vi "Const_uitlity.vi"(1 "Duration":dbl format="%#_13g") -> (0 "Minutes passed":dbl format="%#_13g")   [LabVIEW 2016]
uses:
  Global/Global Variables/Data_Display_global.vi
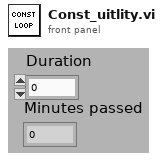
[diagram p1: front panel]
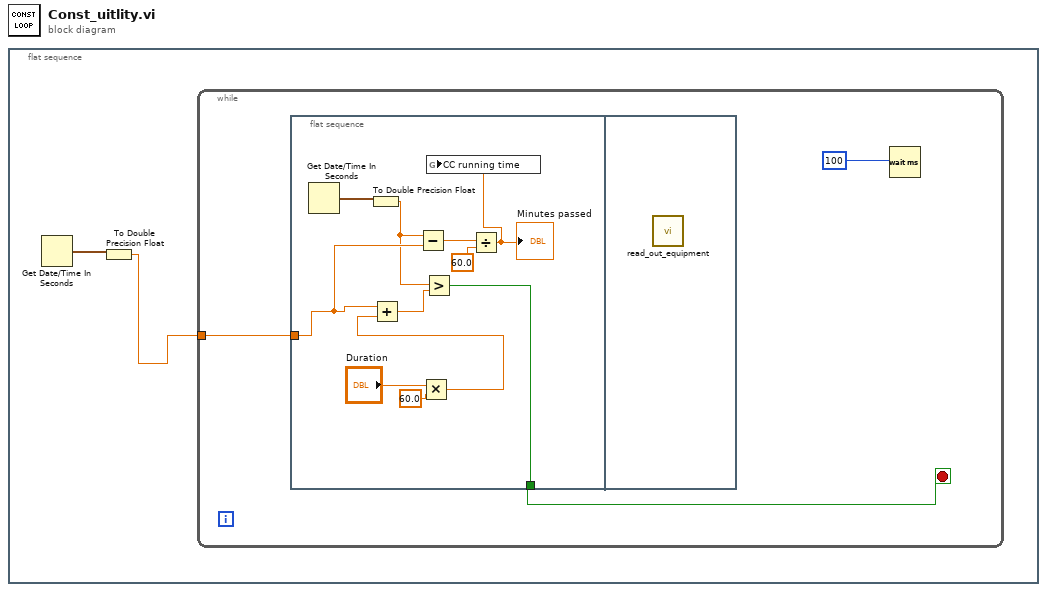
[diagram p0: block diagram]
diagram:
  n1 = flat-sequence {
    frame #0 {
      n2 = Get Date/Time In Seconds() -> (seconds since 1Jan1904=w2:timestamp)
      n3 = To Double Precision Float(number=w2) -> (double precision float=w1:dbl)
      n4 = while {
        tunnel: w1 -> [w4]
        stop <- w5 stop-if-true
        n5 = flat-sequence {
          tunnel: [w12] -> w5
          tunnel: w4 -> [w10]
          frame #0 {
            n6 = Get Date/Time In Seconds() -> (seconds since 1Jan1904=w11:timestamp)
            n7 = To Double Precision Float(number=w11) -> (double precision float=w9:dbl)
            n8 = Subtract(x=w9, y=w10) -> (x-y=w8:dbl)
            n9 = Multiply(x="Duration", y=60.0) -> (x*y=w14:dbl)
            n10 = Add(x=w10, y=w14) -> (x+y=w13:dbl)
            n11 = Greater?(x=w9, y=w13) -> (0:w12:bool)
            n12 = Divide(x=w8, y=60.0) -> (x/y=w6:dbl)
            "Minutes passed" <- w6
            n13 = global write "Data_Display_global.vi" "CC running time"(w6) -> ()
          }
          frame #1 {
            n14 = call "read_out_equipment.vi"() -> ()  [unwired: 1 in]
          }
        }
        n15 = Wait (ms)(milliseconds to wait=100) -> ()  [unwired: 1 out]
      }
    }
  }
